vi "TDMS.HandleFile.vi"(7 "Result Directory":path, 8 "error out":errorcluster, 9 "Delete":bool, 11 "Data":path) -> (0 "error out":errorcluster, 3 "Results Data File":path)   [LabVIEW 2015, in "Analysis.lvlib"]
uses:
  Analysis.lvlib
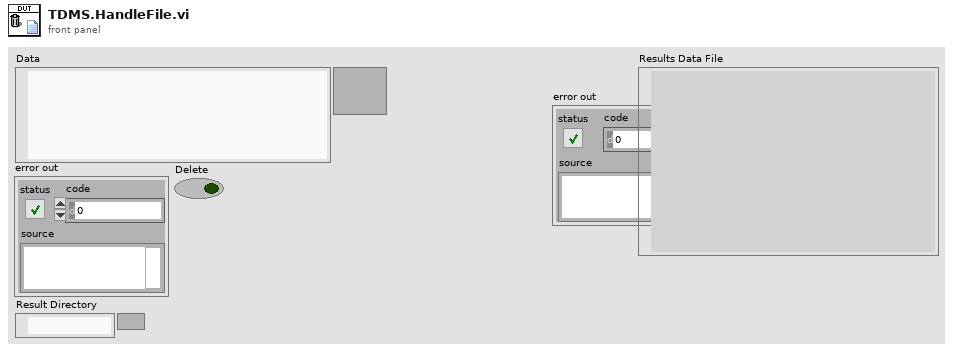
[diagram p1: front panel]
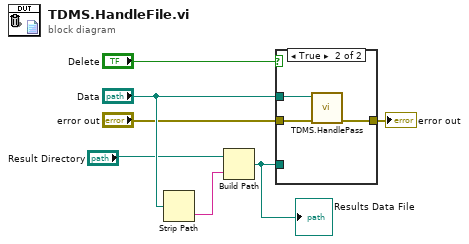
[diagram p0: block diagram]
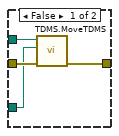
[diagram p2: hidden frame]
diagram:
  n1 = Strip Path(path="Data") -> (name=w1:string)  [unwired: 1 out]
  n2 = Build Path(base path="Result Directory", name or relative path=w1) -> (appended path=w6:path)
  "Results Data File" <- w6
  n3 = case shown="True" "Delete" {
    tunnel: "error out" -> [w11 w14]
    tunnel: [w8 w12] -> w3
    tunnel: "Data" -> [w9 w13]
    tunnel: w6 -> [w10 _]
    frame False {
      n4 = call "TDMS.MoveTDMS.vi"("error in (no error)"=w11, "Target path"=w10, "Source Path"=w9) -> ("error out"=w8:errorcluster)  [unwired: 8 in]
    }
    frame True {
      n5 = call "TDMS.HandlePass.vi"("error in (no error)"=w14, "file path in"=w13) -> ("error out"=w12:errorcluster)  [unwired: 9 in]
    }
  }
  "error out" <- w3
